vi "PID.vi"() -> ()   [LabVIEW 2019]
uses:
  <vilib>/NI/Modbus Library/API/Wrapper/Create Serial Master.vi
  <vilib>/addons/control/pid/pid.llb/PID (DBL).vi
  <vilib>/NI/Modbus Library/API/Master/Modbus Master.lvclass
  <vilib>/NI/Modbus Library/API/Wrapper/API Main.lvlib
  <vilib>/addons/control/pid/NI_PID_pid.lvlib
panel:
  in  "Control de Caragas":T1(ring)
  out "Carga Electrica Automática":dbl
  out "tiempo de control cargas":dbl
  in  "Cargas Automáticas":bool=TRUE
  in  "Cargas Manuales":bool
  out "Señal de control":dbl
  out "Velocidad deseada":dbl
  out "Comportamiento de la planta":dynamicdata(graph)
  out "Frecuencia nueva":dbl
  in  "PID constantes":T2={"proportional gain (Kc)"=1.0, "integral time (Ti, min)"=0.01, "derivative time (Td, min)"=0.0} {"derivative time (Td, min)" format="%.3f"; "integral time (Ti, min)" format="%.3f"; "proportional gain (Kc)" format="%.3f"}
  out "Velocidad deseada automatica":dbl
  in  "Velocidad automática":bool
  out "Tiempo Transcurrido":dbl
  out "Frecuencia de rotación":dbl
  out "Velocidad medida (rpm)":dbl
  in  "Frequency":dbl(knob) step=1.0 scale=0.0..75.0
  in  "VFD":bool
  out "Frecuencia Real VFD":dbl
  in  "stop":bool
  in  "Apagar Ejecución":bool=TRUE
  in  "Baud rate":u32=9600
  in  "Puerto":refnum<visa-resource-name>
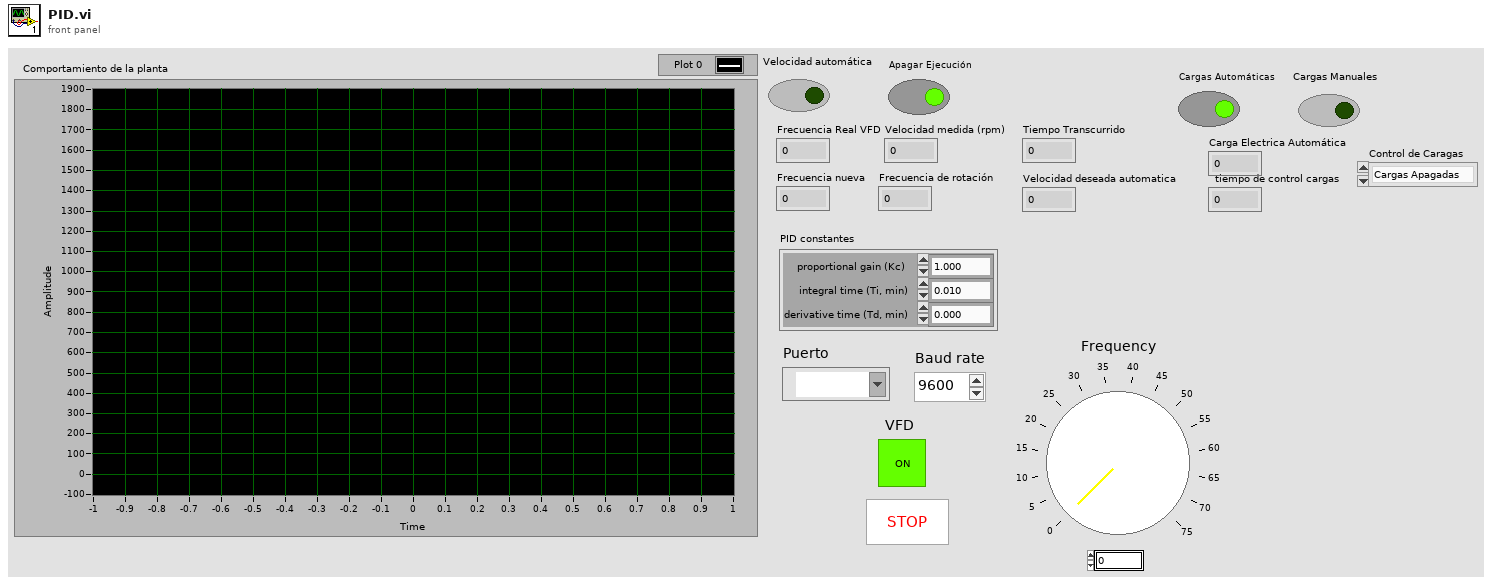
[diagram p1: front panel]
types:
  T1 = enum16{"Cargas Apagadas", "Activar Primer Carga", "Activar Segunda Carga", "Activar Ambas Cargas"}
  T2 = cluster{"proportional gain (Kc)":dbl, "integral time (Ti, min)":dbl, "derivative time (Td, min)":dbl}
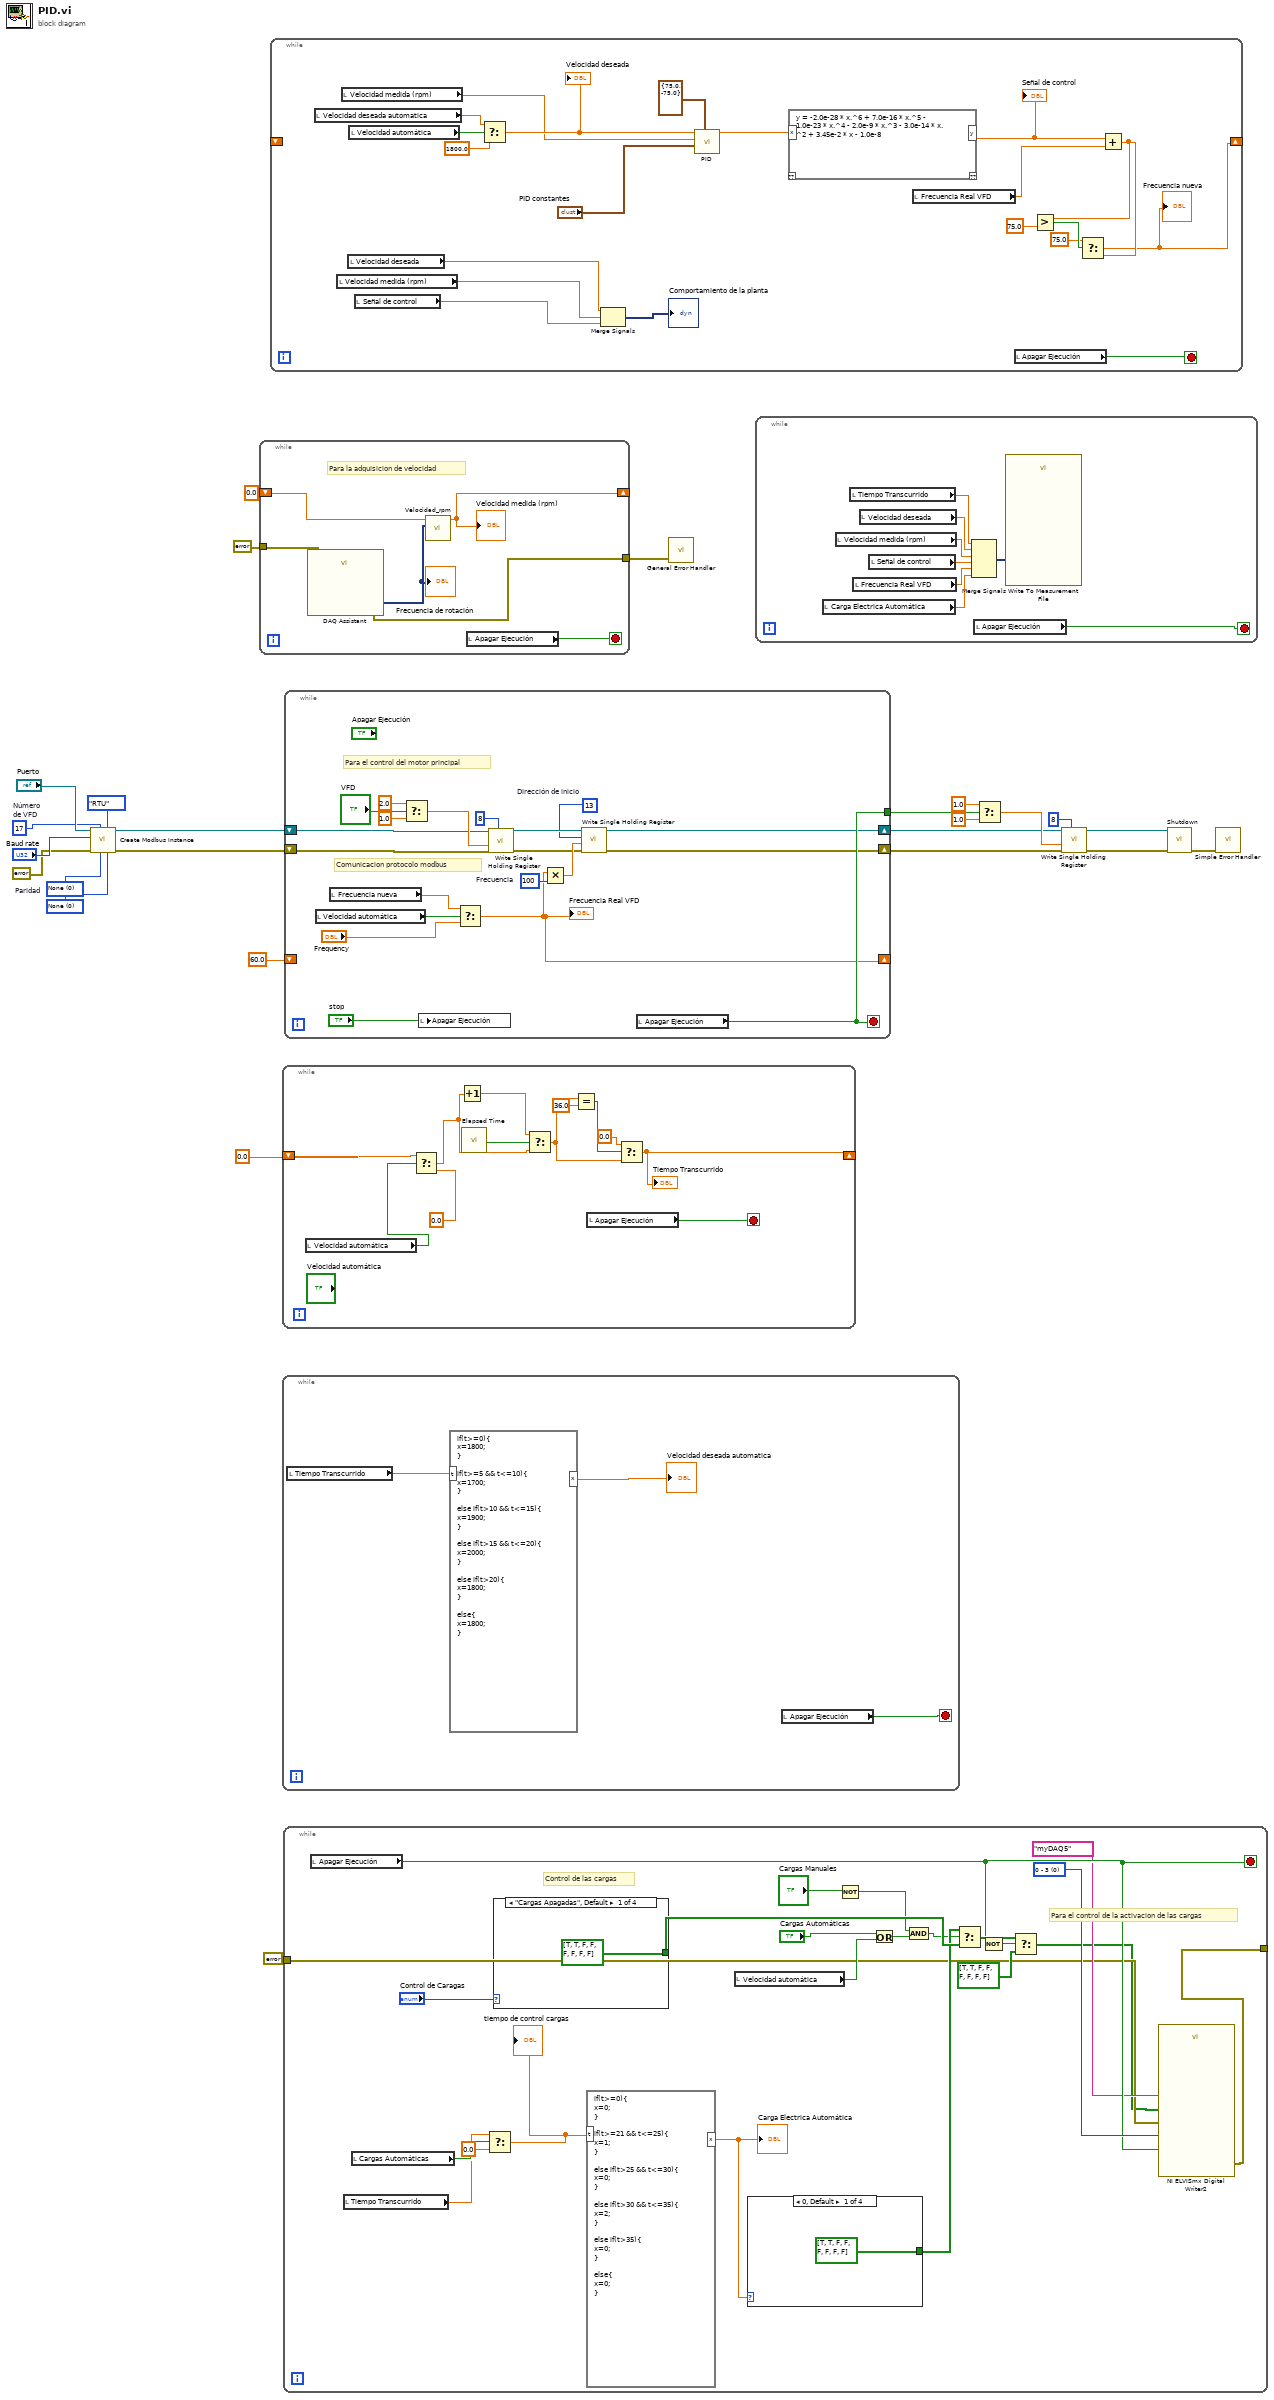
[diagram p0: block diagram]
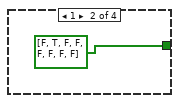
[diagram p2: hidden frame]
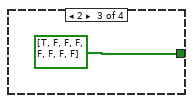
[diagram p3: hidden frame]
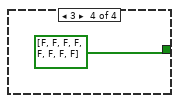
[diagram p4: hidden frame]
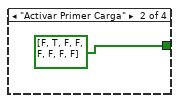
[diagram p5: hidden frame]
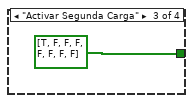
[diagram p6: hidden frame]
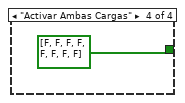
[diagram p7: hidden frame]
diagram:
  w20 = u16 0 items=["None", "Odd", "Even", "Mark", "Space"]  # Paridad
  w21 = u16 0 items=["None", "XON/XOFF", "RTS/CTS", "XON/XOFF & RTS/CTS", "DTR/DSR", "XON/XOFF & DTR/DSR"] ("flow control (none)")
  w19 = u8 17  # Número de VFD
  n1 = call-poly <vilib>:"Create Modbus Instance.vi"("flow control (none)"=w21, "serial type"=enum16{"RTU", "ASCII"}."RTU", "parity (even)"=w20, "unit ID"=w19, "error in"=errorcluster {"status"=FALSE, "code"=0, "source"=""}, "baud rate"="Baud rate", "VISA resource name"="Puerto") -> ("error out"=w10:errorcluster, "serial master instance"=w11:refnum<class "Modbus Master.lvclass">)  [unwired: 3 in]
  n2 = while {
    shift-right: [w30] -> _
    shift-left: 0.0 -> [w31]
    tunnel: [w26] -> w4
    tunnel: errorcluster {"status"=FALSE, "code"=0, "source"=""} ("error in") -> [w28]
    stop <- w29 stop-if-true
    # "Para la adquisicion de velocidad"
    n3 = call "DAQ Assistant"("error in"=w28) -> ("data"=w27:dynamicdata, "error out"=w26:errorcluster)  [unwired: 16 in, 1 out]
    "Frecuencia de rotación" <- w27
    n4 = call "Velocidad_rpm.vi"("data"=w27, "Numeric in"=w31) -> ("Numeric out"=w30:dbl)  [unwired: 9 in]
    "Velocidad medida (rpm)" <- w30
    n5 = local read "Apagar Ejecución"() -> (w29:bool)
  }
  n6 = while {
    shift-right: [w32] -> _
    shift-left: _ -> [_]
    stop <- w41 stop-if-true
    n7 = local read "Velocidad deseada automatica"() -> (w49:dbl)
    n8 = local read "Velocidad medida (rpm)"() -> (w38:dbl)
    n9 = local read "Velocidad medida (rpm)"() -> (w46:dbl)
    n10 = local read "Velocidad deseada"() -> (w39:dbl)
    n11 = local read "Velocidad automática"() -> (w50:bool)
    n12 = local read "Señal de control"() -> (w37:dbl)
    n13 = Select(t=w49, s=w50, f=1800.0) -> (s? t:f=w47:dbl)
    "Velocidad deseada" <- w47
    n14 = Merge Signals(w39, w38, w37) -> (→"Comportamiento de la planta":dynamicdata)
    n15 = call-poly <vilib>:"PID.vi"("output range"=cluster{"output high":dbl, "output low":dbl} {"output high"=75.0, "output low"=-75.0}, "PID gains"="PID constantes", "process variable"=w46, "setpoint"=w47) -> ("output"=w42:dbl)  [unwired: 6 in, 1 out]
    n16 = script code="y = -2.0e-28 * x.^6 + 7.0e-16 * x.^5 - 1.0e-23 * x.^4 - 2.0e-9 * x.^3 - 3.0e-14 * x.^2 + 3.45e-2 * x - 1.0e-8"("x"=w42) -> ("y"=w43:dbl)  [unwired: 1 in, 1 out]
    "Señal de control" <- w43
    n17 = local read "Frecuencia Real VFD"() -> (w44:dbl)
    n18 = local read "Apagar Ejecución"() -> (w41:bool)
    n19 = Add(x=w43, y=w44) -> (x+y=w33:dbl)
    n20 = Greater?(x=w33, y=75.0) -> (0:w35:bool)
    n21 = Select(t=75.0, s=w35, f=w33) -> (s? t:f=w32:dbl)
    "Frecuencia nueva" <- w32
  }
  n22 = while {
    stop <- w54 stop-if-true
    n23 = local read "Tiempo Transcurrido"() -> (w52:dbl)
    n24 = formula code="if(t>=0){\nx=1800;\n}\n\nif(t>=5 && t<=10){\nx=1700;\n}\n\nelse if(t>10 && t<=15){\nx=1900;\n}\n\nelse if(t>15 && t<=20){\nx=2000;\n}\n\nelse if(t>20){\nx=1800;\n}\n\nelse{\nx=1800;\n}"("t"=w52) -> ("x"=→"Velocidad deseada automatica":dbl)
    n25 = local read "Apagar Ejecución"() -> (w54:bool)
  }
  n26 = while {
    shift-right: [w59] -> _
    shift-left: 0.0 ("t") -> [w57]
    stop <- w60 stop-if-true
    n27 = local read "Velocidad automática"() -> (w55:bool)
    n28 = Select(t=w57, s=w55, f=0.0) -> (s? t:f=w58:dbl)
    n29 = Increment(x=w58) -> (x+1=w66:dbl)
    n30 = call "Elapsed Time"() -> ("Time has Elapsed"=w65:bool)  [unwired: 12 in, 7 out]
    n31 = Select(t=w66, s=w65, f=w58) -> (s? t:f=w63:dbl)
    n32 = Equal?(x=w63, y=36.0) -> (x = y?=w64:bool)
    n33 = local read "Apagar Ejecución"() -> (w60:bool)
    n34 = Select(t=0.0, s=w64, f=w63) -> (s? t:f=w59:dbl)
    "Tiempo Transcurrido" <- w59
  }
  n35 = while {
    tunnel: errorcluster {"status"=FALSE, "code"=0, "source"=""} ("error in") -> [w70]
    tunnel: [w74] -> _
    stop <- w72 stop-if-true
    w73 = u16 0 items=["0 - 3", "4 - 7", "0 - 7"] ("myDAQ Lines to Write")
    # "Control de las cargas"
    # "Para el control de la activacion de las cargas"
    n36 = local read "Apagar Ejecución"() -> (w72:bool)
    n37 = local read "Tiempo Transcurrido"() -> (w68:dbl)
    n38 = local read "Cargas Automáticas"() -> (w81:bool)
    n39 = Select(t=w68, s=w81, f=0.0) -> (s? t:f=w82:dbl)
    "tiempo de control cargas" <- w82
    n40 = case shown="\"Cargas Apagadas\", Default" "Control de Caragas" {
      tunnel: [bool[] [TRUE, TRUE, FALSE, FALSE, FALSE, FALSE, FALSE, FALSE] ("DO Lines") bool[] [FALSE, TRUE, FALSE, FALSE, FALSE, FALSE, FALSE, FALSE] ("DO Lines") bool[] [TRUE, FALSE, FALSE, FALSE, FALSE, FALSE, FALSE, FALSE] ("DO Lines") bool[] [FALSE, FALSE, FALSE, FALSE, FALSE, FALSE, FALSE, FALSE] ("DO Lines")] -> w85
      frame "Cargas Apagadas", Default {
      }
      frame "Activar Primer Carga" {
      }
      frame "Activar Segunda Carga" {
      }
      frame "Activar Ambas Cargas" {
      }
    }
    n41 = formula code="if(t>=0){\nx=0;\n}\n\nif(t>=21 && t<=25){\nx=1;\n}\n\nelse if(t>25 && t<=30){\nx=0;\n}\n\nelse if(t>30 && t<=35){\nx=2;\n}\n\nelse if(t>35){\nx=0;\n}\n\nelse{\nx=0;\n}"("t"=w82) -> ("x"=w86:dbl)
    "Carga Electrica Automática" <- w86
    n42 = local read "Velocidad automática"() -> (w80:bool)
    n43 = case shown="0, Default" w86 {
      tunnel: [bool[] [TRUE, TRUE, FALSE, FALSE, FALSE, FALSE, FALSE, FALSE] ("DO Lines") bool[] [FALSE, TRUE, FALSE, FALSE, FALSE, FALSE, FALSE, FALSE] ("DO Lines") bool[] [TRUE, FALSE, FALSE, FALSE, FALSE, FALSE, FALSE, FALSE] ("DO Lines") bool[] [FALSE, FALSE, FALSE, FALSE, FALSE, FALSE, FALSE, FALSE] ("DO Lines")] -> w83
      frame 0, Default {
      }
      frame 1 {
      }
      frame 2 {
      }
      frame 3 {
      }
    }
    n44 = Not(x="Cargas Manuales") -> (.not. x?=w76:bool)
    n45 = Or(x="Cargas Automáticas", y=w80) -> (x .or. y?=w79:bool)
    n46 = And(x=w76, y=w79) -> (x .and. y?=w78:bool)
    n47 = Select(t=w83, s=w78, f=w85) -> (s? t:f=w84:bool[])
    n48 = Not(x=w72) -> (.not. x?=w88:bool)
    n49 = Select(t=w84, s=w88, f=bool[] [TRUE, TRUE, FALSE, FALSE, FALSE, FALSE, FALSE, FALSE] ("DO Lines")) -> (s? t:f=w69:bool[])
    n50 = call "NI ELVISmx Digital Writer2"("Device Name"=tag "myDAQ5", "myDAQ Lines to Write"=w73, "Stop"=w72, "DO Lines"=w69, "error in"=w70) -> ("error out"=w74:errorcluster)  [unwired: 14 in]
  }
  n51 = while {
    shift-right: [w100] -> w8
    shift-left: w11 -> [w107]
    shift-right: [w99] -> w9
    shift-left: w10 -> [w106]
    tunnel: [w105] -> w7
    shift-right: [w98] -> _
    shift-left: 60.0 ("Frequency") -> [_]
    stop <- w105 stop-if-true
    w115 = u16 100  # Frecuencia
    w109 = u16 13  # Dirección de inicio
    # "Comunicacion protocolo modbus"
    # "Para el control del motor principal"
    n52 = local read "Velocidad automática"() -> (w104:bool)
    n53 = local read "Frecuencia nueva"() -> (w103:dbl)
    n54 = Select(t=2.0, s="VFD", f=1.0) -> (s? t:f=w117:dbl)
    n55 = local write "Apagar Ejecución"("stop") -> ()
    n56 = Select(t=w103, s=w104, f="Frequency") -> (s? t:f=w98:dbl)
    "Frecuencia Real VFD" <- w98
    n57 = call-dynamic "Write Single Holding Register.vi"("error in"=w106, "register to write"=w117, "address"=u16 8 ("Start"), "Modbus master in"=w107) -> ("error out"=w111:errorcluster, "Modbus master out"=w110:refnum<class "Modbus Master.lvclass">)  [unwired: 6 in]
    n58 = Multiply(x=w98, y=w115) -> (x*y=w116:dbl)
    n59 = call-dynamic "Write Single Holding Register.vi"("error in"=w111, "register to write"=w116, "address"=w109, "Modbus master in"=w110) -> ("error out"=w99:errorcluster, "Modbus master out"=w100:refnum<class "Modbus Master.lvclass">)  [unwired: 6 in]
    n60 = local read "Apagar Ejecución"() -> (w105:bool)
  }
  n61 = call <vilib>:"General Error Handler.vi"("error in (no error)"=w4) -> ()  [unwired: 10 in, 5 out]
  n62 = while {
    stop <- w125 stop-if-true
    n63 = local read "Carga Electrica Automática"() -> (w118:dbl)
    n64 = local read "Velocidad medida (rpm)"() -> (w121:dbl)
    n65 = local read "Tiempo Transcurrido"() -> (w123:dbl)
    n66 = local read "Frecuencia Real VFD"() -> (w119:dbl)
    n67 = local read "Velocidad deseada"() -> (w122:dbl)
    n68 = local read "Señal de control"() -> (w120:dbl)
    n69 = Merge Signals(w123, w122, w121, w120, w119, w118) -> (w124:dynamicdata)
    n70 = local read "Apagar Ejecución"() -> (w125:bool)
    n71 = call "Write To Measurement File"("Signals"=w124) -> ()  [unwired: 16 in, 3 out]
  }
  n72 = Select(t=1.0, s=w7, f=1.0) -> (s? t:f=w14:dbl)
  n73 = call-dynamic "Write Single Holding Register.vi"("error in"=w9, "register to write"=w14, "address"=u16 8 ("Start"), "Modbus master in"=w8) -> ("error out"=w12:errorcluster, "Modbus master out"=w13:refnum<class "Modbus Master.lvclass">)  [unwired: 6 in]
  n74 = call-dynamic "Shutdown.vi"("error in"=w12, "Modbus master in"=w13) -> ("error out"=w18:errorcluster)  [unwired: 9 in]
  n75 = call <vilib>:"Simple Error Handler.vi"("error in (no error)"=w18) -> ()  [unwired: 4 in, 5 out]
